vi "Hide Window.vi"(0 "Document in":refnum<class "Document.lvclass">, 11 "error in (no error)":errorcluster) -> (4 "Document out":refnum<class "Document.lvclass">, 15 "error out":errorcluster)   [LabVIEW 2016, in "Document.lvclass"]
uses:
  Document.lvclass
  Document.lvclass/Document.ctl
  user32.dll
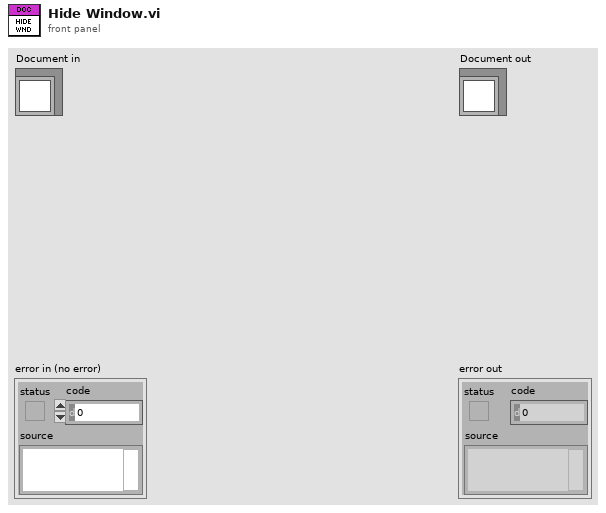
[diagram p1: front panel]
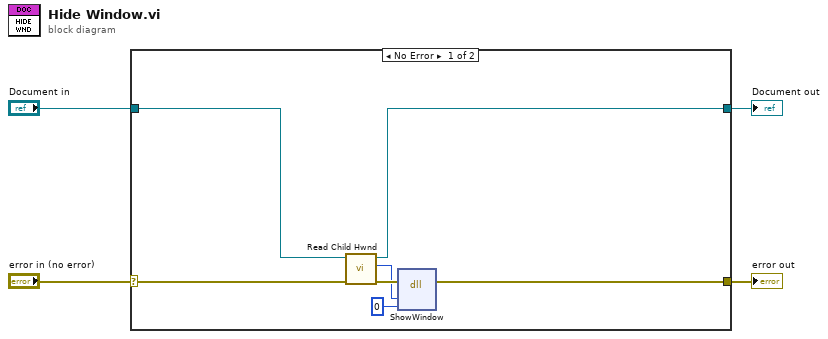
[diagram p0: block diagram]
diagram:
  n1 = case shown="No Error" "error in (no error)" {
    selector: "error in (no error)" -> [w8 w13]
    tunnel: [w7 w13] -> w3
    tunnel: [w5 w12] -> w1
    tunnel: "Document in" -> [w6 w12]
    frame No Error {
      n2 = call "Read Child Hwnd.vi"("error in (no error)"=w8, "Document in"=w6) -> ("error out"=w10:errorcluster, "Child Hwnd"=w9:u32, "Document out"=w5:refnum<class "Document.lvclass">)  [unwired: 7 in]
      n3 = dll-call lib="user32.dll" fn="ShowWindow"(error in=w10, "hwnd"=w9, "nCmdShow"=u32 0) -> (error out=w7:errorcluster)  [unwired: 5 in, 1 out]
    }
    frame Error {
    }
  }
  "error out" <- w3
  "Document out" <- w1
